vi "Save Test Result.vi"(8 "error in (no error)":errorcluster, 10 "Report.lvclass":refnum<class "Report.lvclass">, 11 "Measure in":refnum<class "Measure.lvclass">) -> (0 "error out":errorcluster, 3 "Measure out":refnum<class "Measure.lvclass">)   [LabVIEW 2021, in "Sequence Engine.lvlib" / "Measure.lvclass"]
uses:
  Measure.lvclass
  PPLs/Report.lvlibp/Classes/Report/Report.lvclass
  PPLs/Report.lvlibp/Classes/Report/Test Param.ctl
  Measure.lvclass/Measure.ctl
  Test Result/Test Result.lvclass/Test Result.ctl
  Test Result/Test Result.lvclass
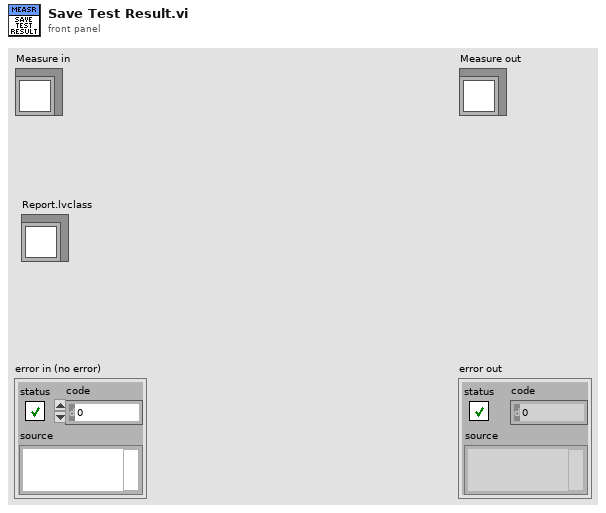
[diagram p1: front panel]
types:
  T1 = typedef "Report.lvlibp/Report.lvclass/Test Param.ctl" = cluster{"Report ID":i32, "Param Name":string, "Expected Value":string, "Value":string, "Test Result":string, "Cycle Time (ms)":dbl}
  T2 = typedef "Sequence Engine.lvlib/Test Result.lvclass/Result Data.ctl" = cluster{"Test ID":u32, "Test Name":string, "Sub Test Name":string, "Test Status":T3, "Start Time":timestamp, "End Time":timestamp, "Duration (s)":dbl, "Expected Values":string, "Measured Values":string, "Remarks":string}
  T3 = typedef "Sequence Engine.lvlib/Test Result.lvclass/Test Status.ctl" = enum16{"Pass", "Fail", "Aborted", "Skipped"}
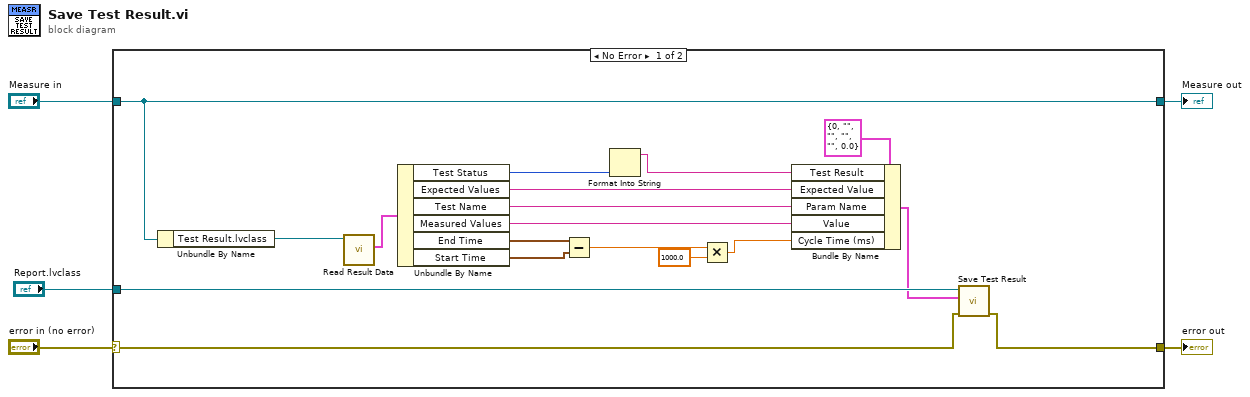
[diagram p0: block diagram]
diagram:
  n1 = case shown="No Error" "error in (no error)" {
    selector: "error in (no error)" -> [w14 w25]
    tunnel: [w13 w25] -> w4
    tunnel: "Measure in" -> [w23 w24]
    tunnel: [w23 w24] -> w2
    tunnel: "Report.lvclass" -> [w22 _]
    frame No Error {
      n2 = Unbundle By Name(w23) -> ("Test Result.lvclass"=w21:refnum<class "Test Result.lvclass">)
      n3 = call "Read Result Data.vi"("Test Result in"=w21) -> ("Result Data"=w20:T2)  [unwired: 8 in, 2 out]
      n4 = Unbundle By Name(w20) -> ("Test Status"=w7:T3, "Expected Values"=w8:string, "Test Name"=w19:string, "Measured Values"=w18:string, "End Time"=w17:timestamp, "Start Time"=w16:timestamp)
      n5 = Subtract(x=w17, y=w16) -> (x-y=w15:dbl)
      n6 = Format Into String(w7) -> (resulting string=w6:string)  [unwired: 3 in, 1 out]
      n7 = Multiply(x=w15, y=1000.0) -> (x*y=w12:dbl)
      n8 = Bundle By Name(cluster=T1 {"Report ID"=0, "Param Name"="", "Expected Value"="", "Value"="", "Test Result"="", "Cycle Time (ms)"=0.0}, "Test Result"=w6, "Expected Value"=w8, "Param Name"=w19, "Value"=w18, "Cycle Time (ms)"=w12) -> (w9:T1)
      n9 = call "Save Test Result.vi"("error in (no error)"=w14, "Test Param"=w9, "Report in"=w22) -> ("error out"=w13:errorcluster)  [unwired: 7 in, 1 out]
    }
    frame Error {
    }
  }
  "error out" <- w4
  "Measure out" <- w2
